vi "AlliGator Build Phasor Ratio Plot Name Prefix.vi"(8 "Error In":errorcluster, 11 "Phasor Plot Name in":string) -> (0 "Error Out":errorcluster, 3 "Phasor Ratio Plot Name Prefix out":string)   [LabVIEW 2021, in "AlliGator Phasor Ratio.lvlib"]
doc: "Strips \" Phasor Plot\" from the source phasor plot name."
uses:
  AlliGator Phasor Ratio.lvlib
panel:
  # "see the AlliGator License on the block diagram (Ctrl+E or Window:Show Block Diagram)"
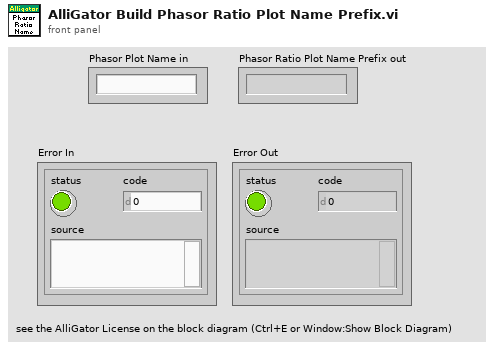
[diagram p1: front panel]
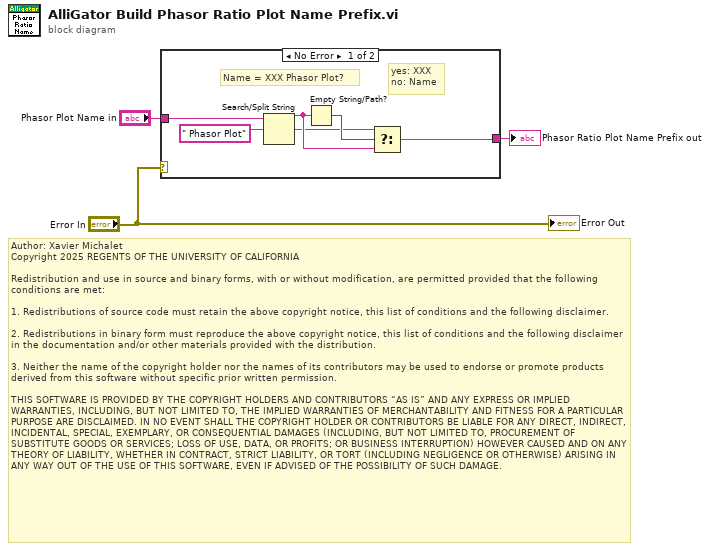
[diagram p0: block diagram]
diagram:
  # "Author: Xavier Michalet\nCopyright 2025 REGENTS OF THE UNIVERSITY OF CALIFORNIA\n\nRedistribution and use in source and binary forms, with or without modification, are permitted provided that the following conditions are met:\n\n1. Redistributions of source code must retain the above copyright notice, this list of conditions and the following disclaimer.\n\n2. Redistributions in binary form must reproduce the above copyright notice, this list of conditions and the following disclaimer in the documentation and/or other materials provided with the distribution.\n\n3. Neither the name of the copyright holder nor the names of its contributors may be used to endorse or promote products derived from this software without specific prior written permission.\n\nTHIS SOFTWARE IS PROVIDED BY THE COPYRIGHT HOLDERS AND CONTRIBUTORS “AS IS” AND ANY EXPRESS OR IMPLIED WARRANTIES, INCLUDING, BUT NOT LIMITED TO, THE IMPLIED WARRANTIES OF MERCHANTABILITY AND FITNESS FOR A PARTICULAR PURPOSE ARE DISCLAIMED. IN NO EVENT SHALL THE COPYRIGHT HOLDER OR CONTRIBUTORS BE LIABLE FOR ANY DIRECT, INDIRECT, INCIDENTAL, SPECIAL, EXEMPLARY, OR CONSEQUENTIAL DAMAGES (INCLUDING, BUT NOT LIMITED TO, PROCUREMENT OF SUBSTITUTE GOODS OR SERVICES; LOSS OF USE, DATA, OR PROFITS; OR BUSINESS INTERRUPTION) HOWEVER CAUSED AND ON ANY THEORY OF LIABILITY, WHETHER IN CONTRACT, STRICT LIABILITY, OR TORT (INCLUDING NEGLIGENCE OR OTHERWISE) ARISING IN ANY WAY OUT OF THE USE OF THIS SOFTWARE, EVEN IF ADVISED OF THE POSSIBILITY OF SUCH DAMAGE."
  n1 = case shown="No Error" "Error In" {
    tunnel: [w4 w10] -> w3
    tunnel: "Phasor Plot Name in" -> [w5 w10]
    frame No Error {
      # "yes: XXX\nno: Name"
      # "Name = XXX Phasor Plot?"
      n2 = Search/Split String(string=w5, search string/char (-)=" Phasor Plot") -> (substring before match=w8:string, match + rest of string=w7:string)  [unwired: 1 in, 1 out]
      n3 = Empty String/Path?(string/path=w8) -> (empty?=w9:bool)
      n4 = Select(t=w7, s=w9, f=w8) -> (s? t:f=w4:string)
    }
    frame Error {
    }
  }
  "Phasor Ratio Plot Name Prefix out" <- w3
  "Error Out" <- "Error In"
